vi "Test Undo Flag.vi"(8 "error in":errorcluster, 11 "History Tests in":refnum<class "History Tests.lvclass">) -> (0 "error out":errorcluster, 3 "History Tests out":refnum<class "History Tests.lvclass">)   [LabVIEW 2020, in "History Tests.lvclass"]
uses:
  History Tests.lvclass
  History Tests.lvclass/History Tests.ctl
  <vilib>/Astemes/LUnit/Test Case.lvclass
  resource/plugins/NIIconEditor/History/History/History.lvclass
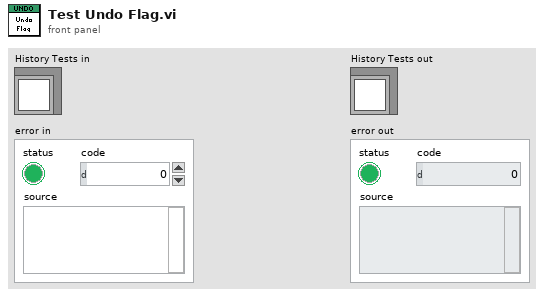
[diagram p1: front panel]
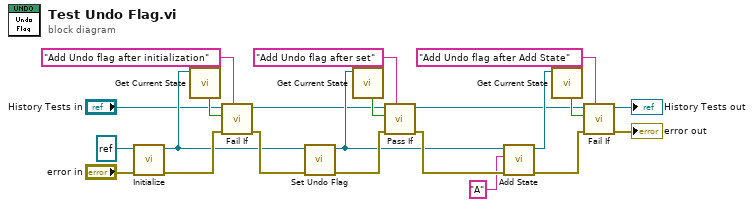
[diagram p0: block diagram]
diagram:
  n1 = call "Initialize.vi"("error in"="error in", "menu reference"=refnum<k9> refnum) -> ("error out"=w18:errorcluster, "History"=w11:refnum<class "History.lvclass">)  [unwired: 8 in]
  n2 = call "Get Current State.vi"("History"=w11) -> ("Add Undo"=w13:bool)  [unwired: 8 in, 2 out]
  n3 = call <vilib>:"Fail If.vi"("Description"="Add Undo flag after initialization", "error in (no error)"=w18, "Fail?"=w13, "LUnit Test Case In"="History Tests in") -> ("error out"=w20:errorcluster, "LUnit Test Case Out"=w2:refnum<class "History Tests.lvclass">)  [unwired: 6 in]
  n4 = call "Set Undo Flag.vi"("error in"=w20, "History in"=w11) -> ("error out"=w17:errorcluster, "History out"=w8:refnum<class "History.lvclass">)  [unwired: 8 in]
  n5 = call "Get Current State.vi"("History"=w8) -> ("Add Undo"=w10:bool)  [unwired: 8 in, 2 out]
  n6 = call <vilib>:"Pass If.vi"("Description"="Add Undo flag after set", "error in (no error)"=w17, "Pass?"=w10, "LUnit Test Case In"=w2) -> ("error out"=w19:errorcluster, "LUnit Test Case Out"=w1:refnum<class "History Tests.lvclass">)  [unwired: 6 in]
  n7 = call "Add State.vi"("error in"=w19, "State"="A", "History in"=w8) -> ("error out"=w16:errorcluster, "History out"=w5:refnum<class "History.lvclass">)  [unwired: 7 in]
  n8 = call "Get Current State.vi"("History"=w5) -> ("Add Undo"=w22:bool)  [unwired: 8 in, 2 out]
  n9 = call <vilib>:"Fail If.vi"("Description"="Add Undo flag after Add State", "error in (no error)"=w16, "Fail?"=w22, "LUnit Test Case In"=w1) -> ("error out"=→"error out":errorcluster, "LUnit Test Case Out"=→"History Tests out":refnum<class "History Tests.lvclass">)  [unwired: 6 in]
